vi "dataProcess_coherenceLength.vi"(0 "reference":refnum<class "OSA300.lvclass">, 1 "samplesPerRefPeriod":i32, 2 "interferogram":sgl[](array[numeric]), 3 "X min interferogram (cm)":sgl, 4 "X max interferogram (cm)":sgl, 5 "error in (no error)":errorcluster, 6 "X range":T1(ring), 8 "X min (cm)":sgl format="%.2f", 10 "X max (cm)":sgl format="%.2f") -> (14 "duplicate reference":refnum<class "OSA300.lvclass">, 15 "coherence length error(cm)":dbl, 16 "coherence length (cm)":dbl, 19 "error out":errorcluster)   [LabVIEW 2010, in "OSA300.lvclass"]
doc: "Estimates the coherence length of the input light source by analyzing the interferogram.\n\nThis vi calls FTS_CoherenceLength_Array, (FTSLib.dll), with the interferogram input parameter pointing to the interferogram control data of this vi or, if empty, to the labview interferogram buffer. \n\nSee buffer_get.vi or trace_toLVBuffer.vi for OSA200 labview buffer handling."
uses:
  OSA300.lvclass
  typeDef/interferogram_properties.ctl
  OSA.lvclass
  FTSLib.dll
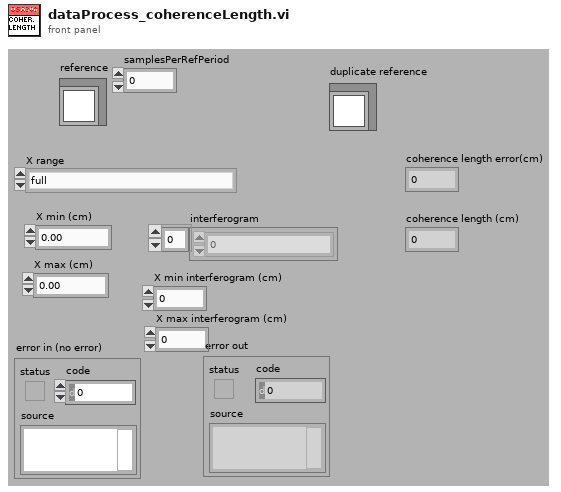
[diagram p1: front panel]
types:
  T1 = enum16{"full", "zero symmetric (-X min .... +X min)", "zero asymmetric (X min .... X max)"}
  T2 = typedef "OSA.lvclass/interferogram_properties.ctl" = cluster{"length":u32, "X min (cm)":sgl, "X max (cm)":sgl, "saturated":bool, "broadband":bool, "isMonoChromatic":bool, "peakToPeak, (counts)":dbl, "peakToPeak position (cm)":dbl, "samplesPerRefPeriod":i32, "OPDmin (cm)":sgl, "OPDmax (cm)":sgl, "contrast (%)":dbl}
  T3 = enum16{"get", "init", "set interferogram", "set spectrum", "cleanUp"}
  T4 = typedef "OSA.lvclass/ObjectAttributes.ctl" = cluster{"Stop":bool, "dataType":T5, "spectrometerIdx":u16, "buffer size interferogram":i32, "interferogram":cluster{"new":bool, "plot_x_ min":sgl, "plot_x_max":sgl, "plot_y_min":sgl, "plot_y_max":sgl, "Graph Intrfrgrm":T6, "timeStamp":u32, "signal (%)":dbl, "traces":cluster{"idx":u32, "broadBand":bool, "monoChromatic":bool, "peakToPeakSignal":dbl, "peakToPeakPos":dbl}[], "traces idx last":i32, "contrast (%)":dbl}, "spectrum":cluster{"new":bool, "plot_x_min":sgl, "plot_x_max":sgl, "plot_unit_x":T7, "plot_unit_y":T8, "plot_y_min":sgl, "plot_y_max":sgl, "Graph Spectrum":T6, "timeStamp":u32, "X_VAL_OPTIONS":enum16{"MIN_MAX", "ARRAY"}, "traces":cluster{"idx":u32}[], "traces idx last":i32}, "Thorlabs_OSA_64.lvclass:queue_action.ctlqueue ref":refnum<queue>, "action":T9, "plot zoom step":dbl, "buffer semaphore":T10, "acq stopped":bool, "dataType active":T5, "temperature (degr C)":sgl, "pressure (hPa)":sgl, "rel humidity (%)":sgl, "settings":cluster{"resolution":u16, "sensitivity":u16, "Average":bool, "average nr":u32, "apodisation":T11, "acq delay (ms)":u32, "airMesure":T12, "wmtr on":bool, "intfgrm_smooth_width":u16, "intfgrm_smooth_nrOfPasses":u16, "intfgrm_smooth":T13, "phaseCorrection":T14, "zeroFill":u8, "spectr_smooth":T13, "spectr_smooth_width":u16, "spectr_smooth_nrOfPasses":u16, "resolution (/cm)":sgl, "REF wavelength, (nm)":dbl, "gain_idx":u16, "gainAuto":bool, "gain_relative":dbl, "PD sensitivity mode":T15, "PD senseMode implemented":bool, "SensorTemperature implemented":bool, "SensorPressure implemented":bool, "SensorHumidity implemented":bool, "attenuationAuto":bool, "attenuationOnOff":bool, "attenuationAvailable":bool, "offsetAvailable":bool, "offset":i32, "offset max":u16, "contrastAvailable":bool}, "peaks position":sgl[], "peaks width":sgl[], "peaks height":sgl[], "peaks max nr":u32, "peaks latest nr":i32, "peaks new":bool, "power":dbl, "power new":bool, "path":string, "wavelength (WNr)":dbl, "wavelength new":bool, "buffer size spectrum":i32, "status":string, "vi reference":refnum<vi>, "funcPointer":u64, "libraryPointer":u64, "singleAcquisition":bool, "coherenceLength (cm)":dbl, "coherenceLength new":bool, "spectrometer model":string, "spectrometer serial nr":string, "peaks thld left":sgl[], "peaks thld right":sgl[], "coherenceLength error (cm)":dbl, "ADC bits":u16, "peaks position centroid":sgl[], "peaks height centroid":sgl[], "OSA series":T16, "channel index spectrum":u16, "spectrometer rangeLow, (/cm)":dbl, "spectrometer rangeHigh, (/cm)":dbl, "channel index interferogram":u16, "virtualSource":bool}
  T5 = typedef "OSA.lvclass/acq_dataType.ctl" = enum16{"none", "interferogram", "spectrum"}
  T6 = typedef "OSA.lvclass/graph_intensity.ctl" = refnum<vi>
  T7 = typedef "OSA.lvclass/spectrum_x_unit.ctl" = enum16{"wavenr/cm", "THz", "eV", "nm_air", "nm_vac"}
  T8 = typedef "OSA.lvclass/y_unit.ctl" = enum16{"ADC counts", "dBm pwr absolute", "dBm pwr density", "mW pwr absolute", "mW pwr density"}
  T9 = typedef "OSA.lvclass/queue_action.ctl" = enum16{"none", "stop", "GUI_plotInterferogram", "GUI_plotSpectrum", "GUI_plotInterferogramRescale", "GUI_plotSpectrumRescale", "GUI_plotInterferogramReset", "GUI_plotSpectrumReset", "GUI_plotInterferogramAutoScaleY", "GUI_plotSpectrumAutoScaleY", "GUI_plotInterferogramZoomOut", "GUI_plotSpectrumZoomOut", "GUI_plotInterferogramPane", "GUI_plotSpectrumPane", "GUI_plotInterferogramZoomMouse", "GUI_plotSpectrumZoomMouse", "GUI_spectrumChannelType", "GUI_channel", "ENVIRONMENT temperature", "ENVIRONMENT pressure", "MODE_resolution set", "MODE_resolution get", "MODE_sensitivity set", "MODE_sensitivity get", "MODE_PDTemperature set", "MODE_PDTemperature get", "REBOOT/RESET firmware", "ACQASYNC_acquireSingleSpectrum", "ACQASYNC_continuous start", "ACQASYNC_continuous stop\n", "ACQASYNC_get last interferogram", "ACQASYNC_get last spectrum", "ACQASYNC_get last waveNr", "ACQOPT_interferogram smoothing set", "ACQOPT_interferogram smoothing get", "ACQOPT_spectrum smoothing set", "ACQOPT_spectrum smoothing get", "ACQOPT_apodisation type set", "ACQOPT_apodisation type get", "ACQOPT_phase correction type set", "ACQOPT_phase correction type get", "ACQOPT_acqIntervall_set", "ACQOPT_acqIntervall_get", "ACQOPT_average spectrum set", "ACQOPT_average spectrum get", "ACQOPT_rolling average set", "ACQOPT_rolling average get", "ACQOPT_zero fill factor set", "ACQOPT_zero fill factor get", "ACQOPT_cycle counting set", "ACQOPT_cycle counting get", "ACQOPT_air measure option set", "ACQOPT_air measure option get", "ACQOPT_gainLevel auto get", "ACQOPT_gainLevel auto set", "ACQOPT_gainLevel get", "ACQOPT_gainLevel set", "ACQOPT_offset set", "ACQOPT_attenuator_auto_set", "ACQOPT_attenuator_set", "ACQOPT_getAll", "INSTRUMENT_PROPERTY_range_WaveNr_min", "INSTRUMENT_PROPERTY_range_WaveNr_max", "INSTRUMENT_PROPERTY_reference_wavelength_cm^-1", "INSTRUMENT_PROPERTY_samplesPerRefPeriod", "INSTRUMENT_PROPERTY_resolution_waveNrPercm", "INSTRUMENT_PROPERTY_availableGainLevels", "INSTRUMENT_PROPERTY_status", "CONVERT", "ANALYSE_POWER", "ANALYSE_PEAKS", "ANALYSE_WAVELENGTH", "ANALYSE_SPECTRUM", "ANALYSE_INTERFEROGRAM", "ANALYSE_COHERENCE_LENGTH", "MATH", "MATH_power", "MATH_peaks", "FILE", "miscellaneous"}
  T10 = typedef "Semaphore RefNum" = refnum<k1>
  T11 = typedef "OSA.lvclass/apodisation.ctl" = enum16{"NONE", "NORTON_BEER_WEAK", "NORTON_BEER_MEDIUM", "NORTON_BEER_STRONG", "TRIANGULAR", "COSINE", "HANN", "HAMMING", "BLACKMANHARRIS3", "BLACKMANHARRIS4", "GAUSSIAN"}
  T12 = typedef "OSA.lvclass/airMeasure.ctl" = enum16{"TEMPERATURE", "PRESSURE"}
  T13 = typedef "OSA20X_misc.lvlib/interferogram_smoothing.ctl" = enum16{"NONE", "BINOMIAL", "SAVITSKY_GOLAY", "FOURIER", "MOVING_AVERAGE", "GAUSSIAN"}
  T14 = typedef "OSA.lvclass/phaseCorrection.ctl" = enum16{"NONE", "MERTZ", "FORMAN", "MERTZ_FILE", "FORMAN_FILE", "FUTURE COMP."}
  T15 = typedef "OSA20X_misc.lvlib/PDTemperatureMode.ctl" = enum16{"cool: better sensitivity/noise floor", "warm: extended wl range"}
  T16 = typedef "OSA.lvclass/OSA_series.ctl" = enum16{"OSA200", "OSA300", "UNKNOWN"}
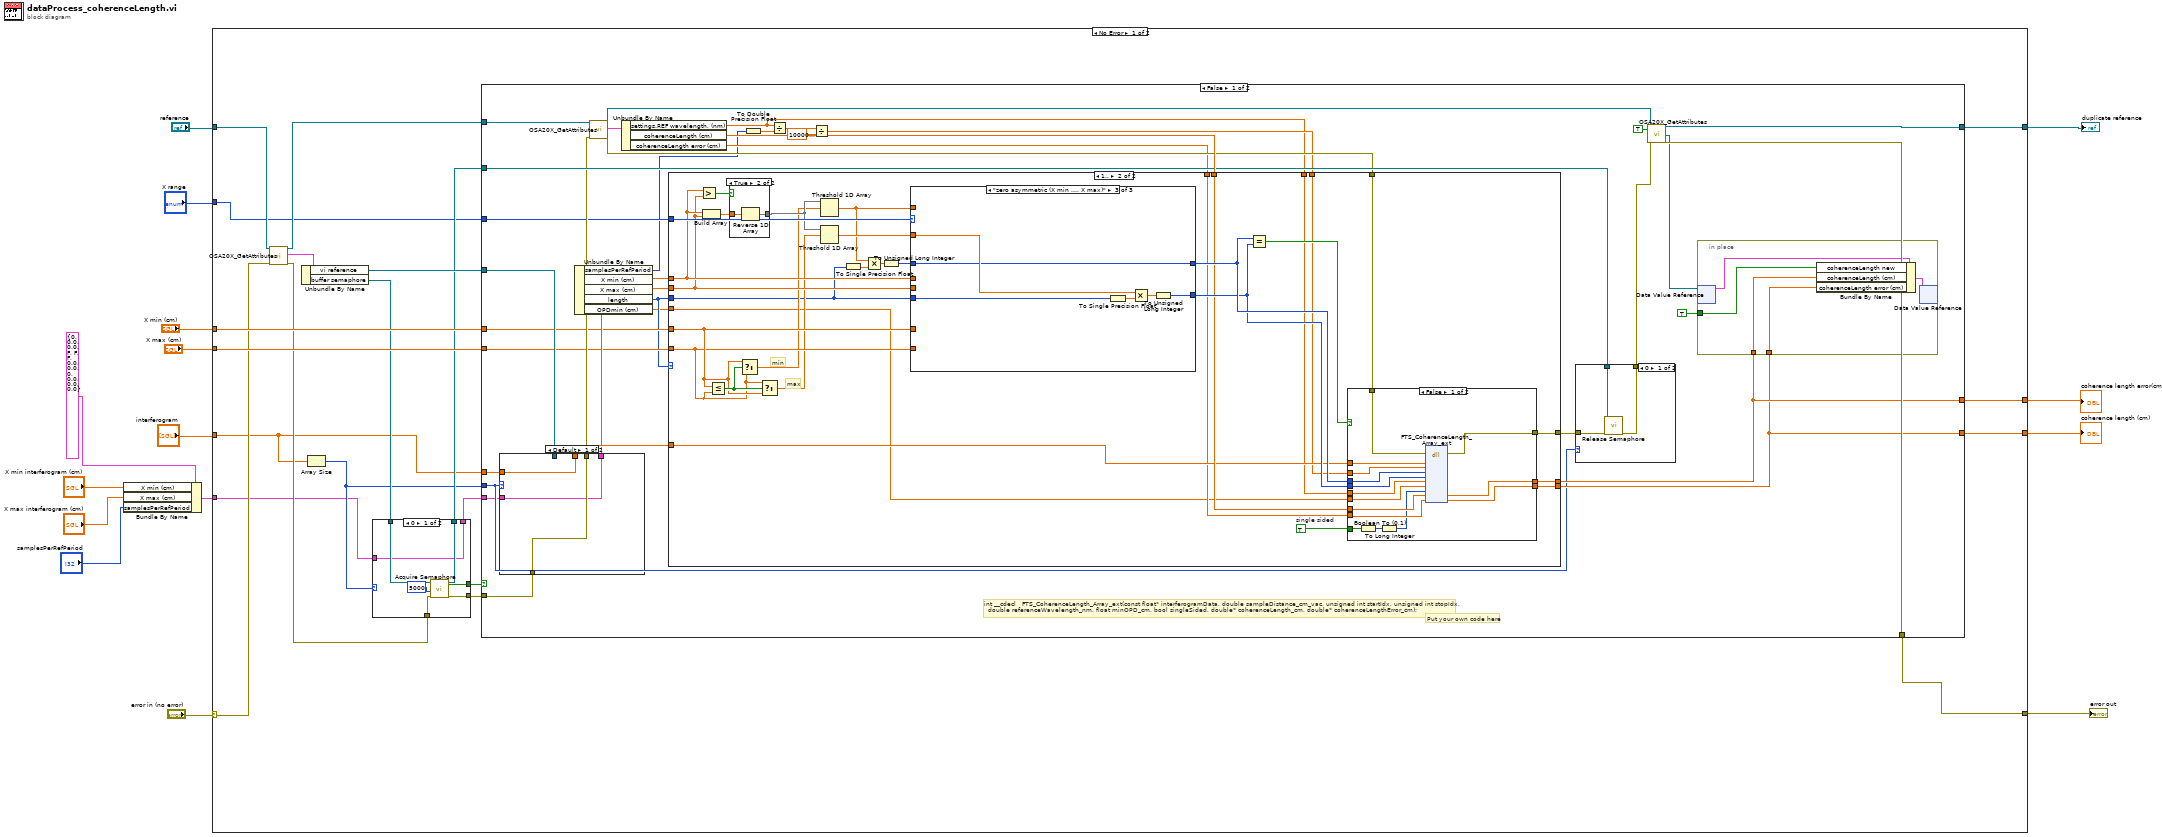
[diagram p0: block diagram]
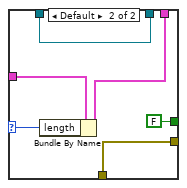
[diagram p2: hidden frame]
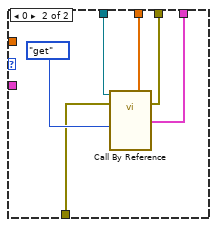
[diagram p4: hidden frame]
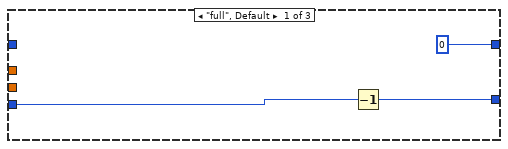
[diagram p7: hidden frame]
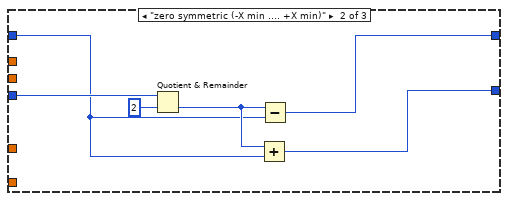
[diagram p8: hidden frame]
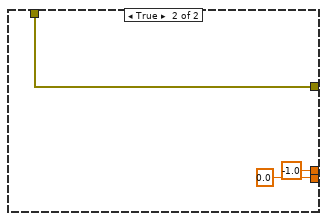
[diagram p9: hidden frame]
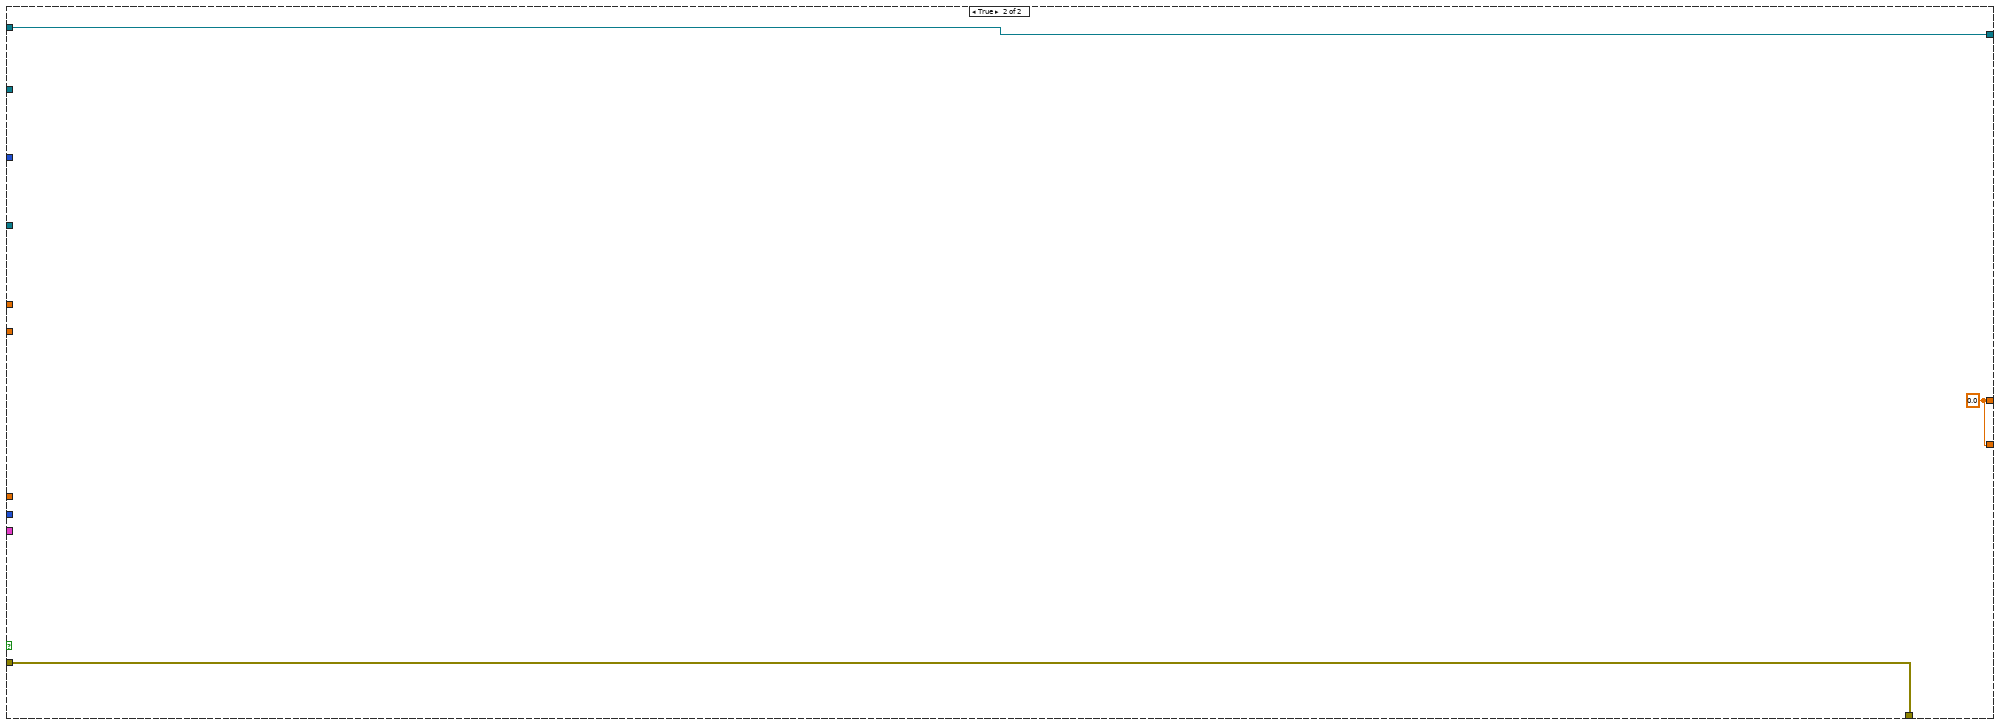
[diagram p10: hidden frame]
diagram:
  n1 = Bundle By Name(cluster=T2 {"length"=0, "X min (cm)"=0.0, "X max (cm)"=0.0, "saturated"=FALSE, "broadband"=FALSE, "isMonoChromatic"=FALSE, "peakToPeak, (counts)"=0.0, "peakToPeak position (cm)"=0.0, "samplesPerRefPeriod"=0, "OPDmin (cm)"=0.0, "OPDmax (cm)"=0.0, "contrast (%)"=0.0} ("interferogram prop set"), "X min (cm)"="X min interferogram (cm)", "X max (cm)"="X max interferogram (cm)", "samplesPerRefPeriod"="samplesPerRefPeriod") -> (w5:T2)
  n2 = case shown="No Error" "error in (no error)" {
    selector: "error in (no error)" -> [w32 w179]
    tunnel: [w35 w179] -> w14
    tunnel: "reference" -> [w26 w180]
    tunnel: [w36 w180] -> w15
    tunnel: "X min (cm)" -> [w34 _]
    tunnel: "X max (cm)" -> [w33 _]
    tunnel: "X range" -> [w22 _]
    tunnel: [w21 w178] -> w12
    tunnel: [w20 w178] -> w13
    tunnel: "interferogram" -> [w19 _]
    tunnel: w5 -> [w17 _]
    frame No Error {
      n3 = call "OSA20X_GetAttributes.vi"("reference in"=w26, "error in (no error)"=w32) -> ("reference out"=w25:refnum<class "OSA300.lvclass">, "Data"=w23:T4, "error out"=w31:errorcluster)  [unwired: 14 in, 1 out]
      n4 = Unbundle By Name(w23) -> ("vi reference"=w27:refnum<vi>, "buffer semaphore"=w29:T10)
      n5 = Array Size(array=w19) -> (size(s)=w18:i32)
      n6 = case shown="0" w18 {
        selector: w18 -> [_ w46]
        tunnel: w31 -> [w42 w48]
        tunnel: [w41 w48] -> w30
        tunnel: w29 -> [w40 w49]
        tunnel: [w39 FALSE ("timed out")] -> w28
        tunnel: [w38 w49] -> w24
        tunnel: w17 -> [w37 w45]
        tunnel: [w37 w44] -> w16
        frame 0 {
          n7 = call <vilib>:"Acquire Semaphore.vi"("error in (no error)"=w42, "ms timeout (-1)"=5000, "semaphore"=w40) -> ("error out"=w41:errorcluster, "timed out"=w39:bool, "semaphore out"=w38:T10)  [unwired: 2 in]
        }
        frame Default {
          n8 = Bundle By Name(cluster=w45, "length"=w46) -> (w44:T2)
        }
      }
      n9 = case shown="False" w28 {
        tunnel: w25 -> [w86 w177]
        tunnel: [w84 w177] -> w36
        tunnel: [w83 w176] -> w35
        tunnel: w34 -> [w63 _]
        tunnel: w33 -> [w62 _]
        tunnel: w30 -> [w81 w176]
        tunnel: w27 -> [w80 _]
        tunnel: w24 -> [w77 _]
        tunnel: w22 -> [w67 _]
        tunnel: [w60 w175] -> w21
        tunnel: [w59 w175] -> w20
        tunnel: w18 -> [w54 _]
        tunnel: w19 -> [w55 _]
        tunnel: w16 -> [w53 _]
        frame False {
          # "int __cdecl   FTS_CoherenceLength_Array_ext(const float* interferogramData, double sampleDistance_cm_vac, unsigned int startIdx, unsigned int stopIdx,  \n\t\tdouble referenceWavelength_nm, float minOPD_cm, bool singleSided, double* coherenceLength_cm, double* coherenceLengthError_cm);"
          # "Put your own code here"
          n10 = case shown="Default" w54 {
            tunnel: w81 -> [w92 w98]
            tunnel: w80 -> [_ w97]
            tunnel: [w92 w96] -> w76
            tunnel: [w93 w95] -> w70
            tunnel: [w91 w94] -> w66
            tunnel: w55 -> [w93 _]
            tunnel: w53 -> [w91 _]
            frame Default {
            }
            frame 0 {
              n11 = call-by-ref "?"(reference=w97, error in=w98, "action"=T3."get") -> (error out=w96:errorcluster, "interferogram"=w95:sgl[], "interferogram prop"=w94:T2)  [unwired: 14 in, 4 out]
            }
          }
          n12 = Unbundle By Name(w66) -> ("samplesPerRefPeriod"=w52:i32, "X min (cm)"=w65:sgl, "X max (cm)"=w64:sgl, "length"=w61:u32, "OPDmin (cm)"=w50:sgl)
          n13 = call "OSA20X_GetAttributes.vi"("reference in"=w86, "error in (no error)"=w76) -> ("reference out"=w85:refnum<class "OSA300.lvclass">, "Data"=w74:T4, "error out"=w71:errorcluster)  [unwired: 14 in, 1 out]
          n14 = Unbundle By Name(w74) -> ("settings.REF wavelength, (nm)"=w51:dbl, "coherenceLength (cm)"=w82:dbl, "coherenceLength error (cm)"=w68:dbl)
          n15 = To Double Precision Float(number=w52) -> (double precision float=w69:dbl)
          n16 = Divide(x=w51, y=w69) -> (x/y=w58:dbl)
          n17 = Divide(x=w58, y=10000000.0) -> (x/y=w56:dbl)
          n18 = case shown="1.." w61 {
            tunnel: w82 -> [w101 w130]
            tunnel: [w100 w129] -> w79
            tunnel: w71 -> [w100 w128]
            tunnel: w70 -> [_ w127]
            tunnel: w56 -> [_ w126]
            tunnel: [w101 w125] -> w60
            tunnel: [w102 w124] -> w59
            tunnel: w68 -> [w102 w123]
            tunnel: w67 -> [_ w122]
            tunnel: w65 -> [_ w118]
            tunnel: w64 -> [_ w117]
            tunnel: w63 -> [_ w115]
            tunnel: w62 -> [_ w114]
            tunnel: w61 -> [_ w108]
            tunnel: w51 -> [_ w105]
            tunnel: w50 -> [_ w104]
            frame 0, Default {
            }
            frame 1.. {
              w103 = TRUE  # single sided
              # "max"
              # "min"
              n19 = Greater?(x=w118, y=w117) -> (0:w120:bool)
              n20 = Build Array(w118, w117) -> (w121:sgl[])
              n21 = Less Or Equal?(x=w115, y=w114) -> (x <= y?=w116:bool)
              n22 = case shown="True" w120 {
                tunnel: w121 -> [w134 w136]
                tunnel: [w134 w135] -> w119
                frame False {
                }
                frame True {
                  n23 = Reverse 1D Array(array=w136) -> (reversed array=w135:sgl[])
                }
              }
              n24 = Select(t=w115, s=w116, f=w114) -> (s? t:f=w113:sgl)
              n25 = Select(t=w114, s=w116, f=w115) -> (s? t:f=w112:sgl)
              n26 = Threshold 1D Array(2:w113, 3:w119) -> (0:w109:sgl)  [unwired: 1 in]
              n27 = Threshold 1D Array(2:w112, 3:w119) -> (0:w111:sgl)  [unwired: 1 in]
              n28 = To Single Precision Float(number=w108) -> (single precision float=w110:sgl)
              n29 = Multiply(x=w109, y=w110) -> (x*y=w107:sgl)
              n30 = To Unsigned Long Integer(number=w107) -> (unsigned 32bit integer=w106:u32)
              n31 = case shown="\"zero asymmetric (X min .... X max)\"" w122 {
                tunnel: w115 -> [_ _ _]
                tunnel: w114 -> [_ _ _]
                tunnel: [u32 0 w141 w146] -> w133
                tunnel: [w138 w140 w149] -> w132
                tunnel: w118 -> [_ _ _]
                tunnel: w117 -> [_ _ _]
                tunnel: w108 -> [w137 w145 w148]
                tunnel: w109 -> [_ _ _]
                tunnel: w111 -> [_ _ w147]
                tunnel: w106 -> [_ w142 w146]
                frame "full", Default {
                  n32 = Decrement(x=w137) -> (x-1=w138:u32)
                }
                frame "zero symmetric (-X min .... +X min)" {
                  n33 = Quotient & Remainder(x=w145, y=u32 2) -> (floor(x/y)=w143:u32)  [unwired: 1 out]
                  n34 = Add(x=w143, y=w142) -> (x+y=w140:u32)
                  n35 = Subtract(x=w143, y=w142) -> (x-y=w141:u32)
                }
                frame "zero asymmetric (X min .... X max)" {
                  n36 = To Single Precision Float(number=w148) -> (single precision float=w151:sgl)
                  n37 = Multiply(x=w147, y=w151) -> (x*y=w150:sgl)
                  n38 = To Unsigned Long Integer(number=w150) -> (unsigned 32bit integer=w149:u32)
                }
              }
              n39 = Equal?(x=w133, y=w132) -> (x = y?=w131:bool)
              n40 = case shown="False" w131 {
                tunnel: w130 -> [w161 _]
                tunnel: w127 -> [w164 _]
                tunnel: w133 -> [w163 _]
                tunnel: w132 -> [w162 _]
                tunnel: [w165 w169] -> w129
                tunnel: w128 -> [w166 w169]
                tunnel: w126 -> [w160 _]
                tunnel: [w159 -1.0 ("coherenceLength")] -> w125
                tunnel: [w158 0.0 ("coherenceLength_error")] -> w124
                tunnel: w123 -> [w157 _]
                tunnel: w105 -> [w156 _]
                tunnel: w104 -> [w155 _]
                tunnel: w103 -> [w154 _]
                frame False {
                  n41 = Boolean To (0,1)(Boolean=w154) -> (0, 1=w153:i16)
                  n42 = To Long Integer(number=w153) -> (32bit integer=w152:i32)
                  n43 = dll-call lib="FTSLib.dll" fn="FTS_CoherenceLength_Array_ext"(error in=w166, "intrfgrm"=w164, "sampleDist_cm_vac"=w160, "idxStart"=w163, "idxStop"=w162, "referenceWave_nm"=w156, "minOPD"=w155, "singleSided_bool"=w152, "coherenceLength"=w161, "coherenceLength_error"=w157) -> (error out=w165:errorcluster, "coherenceLength"=w159:dbl, "coherenceLength_error"=w158:dbl)  [unwired: 10 in, 1 out]
                }
                frame True {
                }
              }
            }
          }
          n44 = case shown="0" w54 {
            tunnel: w79 -> [w89 w90]
            tunnel: [w88 w90] -> w78
            tunnel: w77 -> [w87 _]
            frame 0 {
              n45 = call <vilib>:"Release Semaphore.vi"("error in (no error)"=w89, "semaphore"=w87) -> ("error out"=w88:errorcluster)  [unwired: 4 in, 1 out]
            }
            frame Default {
            }
          }
          n46 = call "OSA20X_GetAttributes.vi"("reference in"=w85, "OnlyGetDvrReference(False)"=TRUE, "error in (no error)"=w78) -> ("reference out"=w84:refnum<class "OSA300.lvclass">, "DataRef"=w73:refnum<data-value>, "error out"=w83:errorcluster)  [unwired: 13 in, 1 out]
          n47 = in-place {
            in-place-border: TRUE ("peaks new") -> [w173]
            in-place-border: w60 -> [w171]
            in-place-border: w59 -> [w170]
            n48 = in-place-dvr #1(w73) -> (w174:T4)  [unwired: 1 out]
            n49 = Bundle By Name(cluster=w174, "coherenceLength new"=w173, "coherenceLength (cm)"=w171, "coherenceLength error (cm)"=w170) -> (w172:T4)
            n50 = in-place-dvr #1(w172) -> ()  [unwired: 2 out]
          }
        }
        frame True {
          w175 = 0.0 ("coherenceLength")
        }
      }
    }
    frame Error {
      w178 = 0.0 ("coherenceLength")
      # "Error"
    }
  }
  "error out" <- w14
  "duplicate reference" <- w15
  "coherence length error(cm)" <- w12
  "coherence length (cm)" <- w13
